vi "IMAQReadMultiMetadata.vi"(8 "error in (no error)":errorcluster, 9 "Keys":string[](array[string]), 10 "Image In":T1, 11 "GRMActor in":refnum<class "GeneralRMActor.lvclass">) -> (0 "error out":errorcluster, 1 "Values":string[](array[string]), 2 "Image Out":T1, 3 "GRMActor out":refnum<class "GeneralRMActor.lvclass">)   [LabVIEW 2020, in "GeneralRMActor.lvlib" / "GeneralRMActor.lvclass"]
uses:
  GeneralRMActor.lvclass
  <vilib>/vision/Image Controls.llb/IMAQ Image.ctl
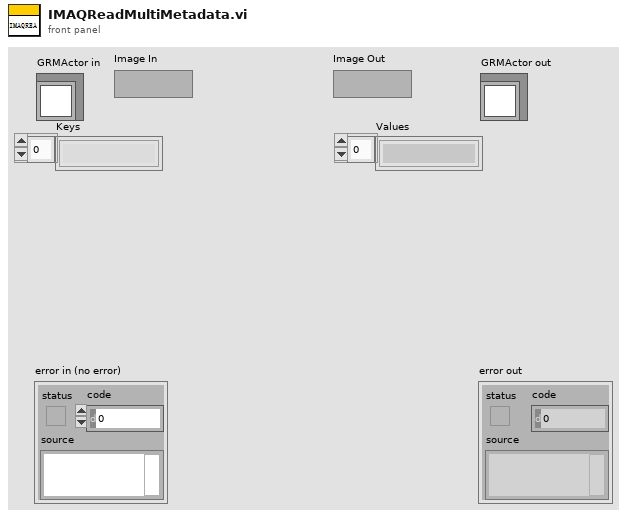
[diagram p1: front panel]
types:
  T1 = typedef "IMAQ Image.ctl" = refnum<image>
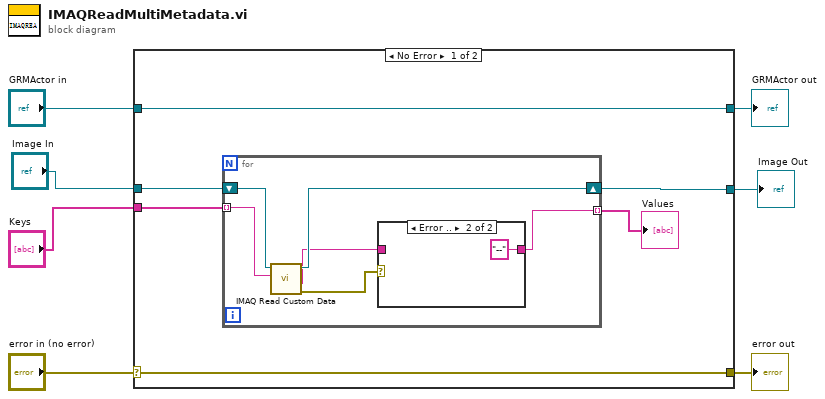
[diagram p0: block diagram]
diagram:
  n1 = case shown="No Error" "error in (no error)" {
    selector: "error in (no error)" -> [w12 w24]
    tunnel: [w12 w24] -> w6
    tunnel: [w13 w23] -> w4
    tunnel: "GRMActor in" -> [w13 w23]
    tunnel: "Image In" -> [w11 w22]
    tunnel: "Keys" -> [w10 _]
    tunnel: [w9 w22] -> w1
    frame No Error {
      n2 = for {
        tunnel: w10 -> [w17] mode=indexing
        shift-right: [w18] -> w9
        shift-left: w11 -> [w19]
        tunnel: [w14] -> w8 mode=indexing
        n3 = call "IMAQ Read Custom Data"("Key"=w17, "Image"=w19) -> ("error out"=w16:errorcluster, "Custom Data Out"=w15:string, "Image (duplicate)"=w18:T1)  [unwired: 7 in]
        n4 = case shown="Error .." w16 {
          tunnel: w15 -> [w20 _]
          tunnel: [w20 "--" ("Custom Data Out")] -> w14
          frame No Error {
          }
          frame Error {
          }
        }
      }
      "Values" <- w8
    }
    frame Error {
    }
  }
  "error out" <- w6
  "GRMActor out" <- w4
  "Image Out" <- w1
